vi "cDAQ Digitize.vi"(8 "error in":errorcluster, 10 "N":i32, 11 "cdaq session in":T1={"mclk [Hz]"=12800000.0, "ADC task"="", "mclk reference"="", "fs [Hz]"=50000.0, "queue adc cmd"=refnum, "queue adc data"=refnum, "adc proc ref"=refnum, "channels"=[], "last channels"=[], "timeout"=timestamp(0 s since 1904-01-01), "N"=1000, "mclk mode"=enum."Free running", "ext mclk source"=""} {"last channels"."Channel id" min=0 step=1; "channels"."Channel id" min=0 step=1}) -> (0 "error out":errorcluster, 3 "cdaq session out":T1={"mclk [Hz]"=12800000.0, "ADC task"="", "mclk reference"="", "fs [Hz]"=50000.0, "queue adc cmd"=refnum, "queue adc data"=refnum, "adc proc ref"=refnum, "channels"=[], "last channels"=[], "timeout"=timestamp(0 s since 1904-01-01), "N"=1000, "mclk mode"=enum."Free running", "ext mclk source"=""} {"last channels"."Channel id" min=0 step=1; "channels"."Channel id" min=0 step=1})   [LabVIEW 2020]
uses:
  cDAQ Session.ctl
  low_level_old/cdaq_anal_adc_command.ctl
  low_level_old/cdaq_anal_adc_data.ctl
  cDAQ Virtual Channel.ctl
  cDAQ Master Clock Mode.ctl
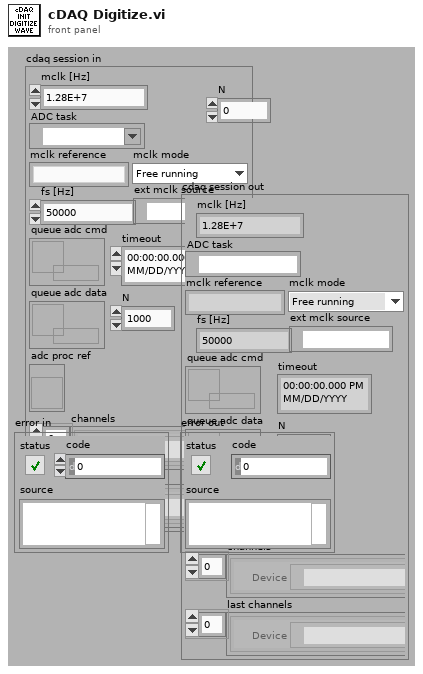
[diagram p1: front panel]
types:
  T1 = typedef "cDAQ Session.ctl" = cluster{"mclk [Hz]":dbl, "ADC task":refnum<k21>, "mclk reference":string, "fs [Hz]":dbl, "queue adc cmd":refnum<queue>, "queue adc data":refnum<queue>, "adc proc ref":refnum<vi>, "channels":T2[], "last channels":T2[], "timeout":timestamp, "N":i32, "mclk mode":T3, "ext mclk source":tag}
  T2 = typedef "cDAQ Virtual Channel.ctl" = cluster{"Device":tag, "Channel id":i32, "btn clr":bool, "btn up":bool, "btn down":bool}
  T3 = typedef "cDAQ Master Clock Mode.ctl" = enum16{"Free running", "Export master clock", "Import master clock"}
  T4 = typedef "cdaq_anal_adc_command.ctl" = cluster{"sample to get":i32, "stop":bool, "abort":bool}
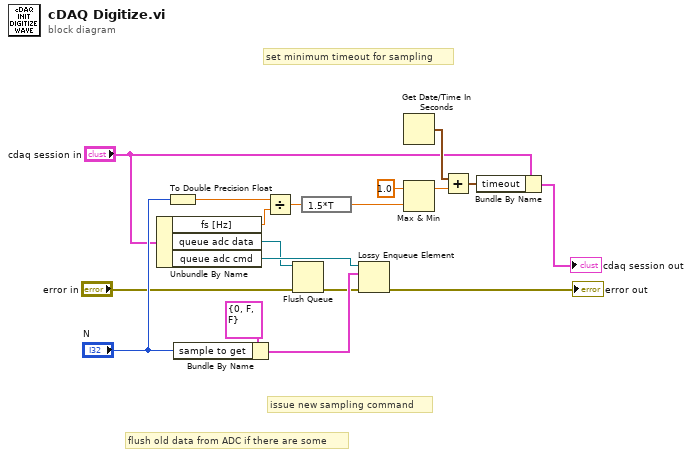
[diagram p0: block diagram]
diagram:
  # "set minimum timeout for sampling"
  # "issue new sampling command"
  # "flush old data from ADC if there are some"
  n1 = Unbundle By Name("cdaq session in") -> ("fs [Hz]"=w13:dbl, "queue adc data"=w9:refnum<queue>, "queue adc cmd"=w17:refnum<queue>)
  n2 = To Double Precision Float(number="N") -> (double precision float=w14:dbl)
  n3 = Bundle By Name(cluster=T4 {"sample to get"=0, "stop"=FALSE, "abort"=FALSE} ("adc cmd"), "sample to get"="N") -> (w16:T4)
  n4 = Divide(x=w14, y=w13) -> (x/y=w12:dbl)
  n5 = Flush Queue(queue=w9, error in (no error)="error in") -> (error out=w11:errorcluster)  [unwired: 2 out]
  n6 = expression code="1.5*T"(w12) -> (w7:dbl)
  n7 = Lossy Enqueue Element(queue=w17, element=w16, error in (no error)=w11) -> (error out=→"error out":errorcluster)  [unwired: 3 out]
  n8 = Get Date/Time In Seconds() -> (seconds since 1Jan1904=w5:timestamp)
  n9 = Max & Min(x=1.0, y=w7) -> (max(x,y)=w6:dbl)  [unwired: 1 out]
  n10 = Add(x=w5, y=w6) -> (x+y=w1:timestamp)
  n11 = Bundle By Name(cluster="cdaq session in", "timeout"=w1) -> (→"cdaq session out":T1)
